vi "Find Value from Key.vi"(8 "error in (no error)":errorcluster, 10 "key":string, 11 "JSON Object in":refnum<class "JSON Object.lvclass">) -> (0 "error out":errorcluster, 2 "value":refnum<class "JSON Datatype.lvclass">)   [LabVIEW 2017, in "LVJSON.lvlib" / "JSON Object.lvclass"]
uses:
  JSON Object.lvclass
  JSON Datatype/JSON Datatype.lvclass
  JSON Object.lvclass/JSON Object.ctl
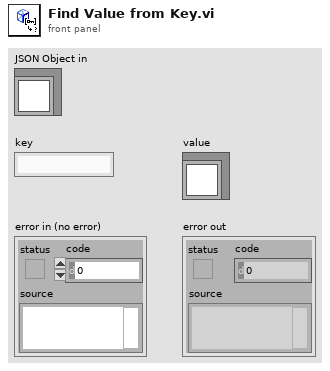
[diagram p1: front panel]
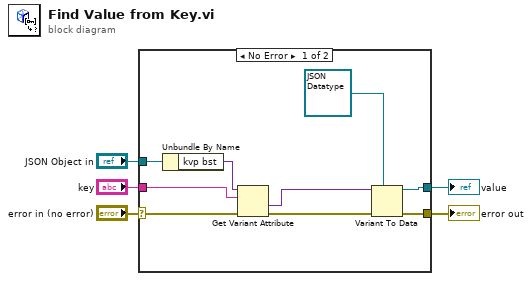
[diagram p0: block diagram]
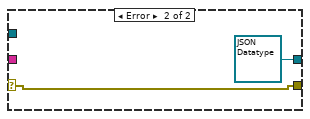
[diagram p2: hidden frame]
diagram:
  n1 = case shown="No Error" "error in (no error)" {
    selector: "error in (no error)" -> [w11 w16]
    tunnel: [w9 w16] -> w4
    tunnel: "JSON Object in" -> [w14 _]
    tunnel: "key" -> [w13 _]
    tunnel: [w7 refnum<class "JSON Datatype.lvclass"> refnum ("value")] -> w1
    frame No Error {
      n2 = Unbundle By Name(w14) -> ("kvp bst"=w6:variant)
      n3 = Get Variant Attribute(Variant=w6, name=w13, error in=w11) -> (value=w12:variant, error out=w10:errorcluster)  [unwired: 1 in, 2 out]
      n4 = Variant To Data(error in=w10, type=refnum<class "JSON Datatype.lvclass"> refnum ("JSON Datatype.lvclass"), Variant=w12) -> (data=w7:refnum<class "JSON Datatype.lvclass">, error out=w9:errorcluster)
    }
    frame Error {
    }
  }
  "error out" <- w4
  "value" <- w1
